vi "Joystick 2 ClimbSystem.vi"(9 "Range of motion":dbl=90.0 format="%#_13g", 10 "Secondary Joystick Buttons":bool[](array[boolean]), 11 "Secondary Joystick Values":dbl[](array[numeric])) -> (2 "Reset Climber Encoder":bool, 3 "Desired Climber Angle":dbl)   [LabVIEW 2018]
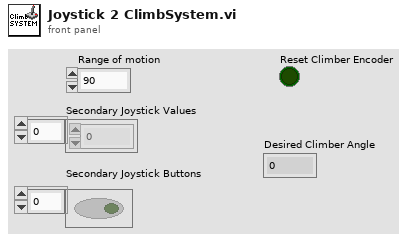
[diagram p1: front panel]
types:
  T1 = typedef "SecondaryJoystickButtons.ctl" = cluster{"Intake":bool, "Outtake":bool, "Arm Up":bool, "Arm Down":bool, "Open Grip":bool, "Close Grip":bool, "Climber Up":bool, "Climber Down":bool, "Reset Climber Encoder":bool}
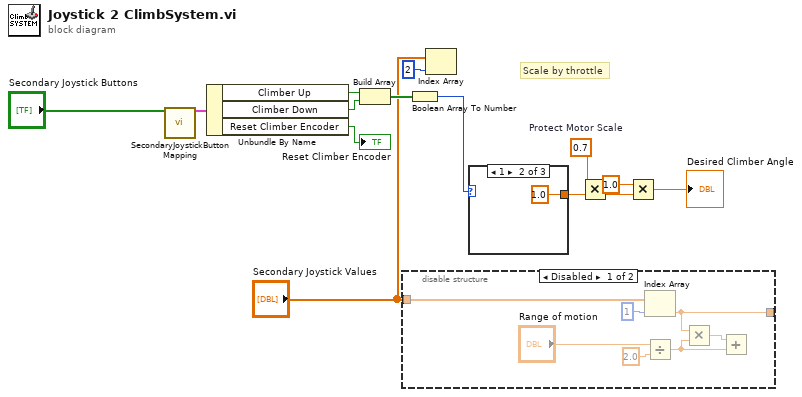
[diagram p0: block diagram]
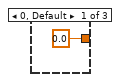
[diagram p2: hidden frame]
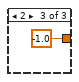
[diagram p3: hidden frame]
diagram:
  w2 = 0.7  # Protect Motor Scale
  # "Scale by throttle"
  n1 = call "SecondaryJoystickButtonMapping.vi"("Secondary joystick buttons"="Secondary Joystick Buttons") -> ("SecondaryJoystickButtons"=w13:T1)  [unwired: 13 in, 1 out]
  n2 = Unbundle By Name(w13) -> ("Climber Up"=w11:bool, "Climber Down"=w10:bool, "Reset Climber Encoder"=→"Reset Climber Encoder":bool)
  n3 = Build Array(w11, w10) -> (w9:bool[])
  n4 = disable-structure shown="Disabled" {
    disable-tunnel: [w16 _] -> _
    disable-tunnel: "Secondary Joystick Values" -> [w15 _]
    frame Disabled {
      n5 = Index Array(array=w15, index=1) -> (element=w16:dbl)
      n6 = Divide(x="Range of motion", y=2.0) -> (x/y=w18:dbl)
      n7 = Multiply(x=w16, y=w18) -> (x*y=w20:dbl)
      n8 = Add(x=w20, y=w18) -> ()  [unwired: 1 out]
    }
    frame Enabled {
    }
  }
  n9 = Boolean Array To Number(Boolean array=w9) -> (number=w8:u32)
  n10 = Index Array(array="Secondary Joystick Values", index=2) -> ()  [unwired: 1 out]
  n11 = case shown="1" w8 {
    tunnel: [0.0 1.0 -1.0] -> w7
    frame 0, Default {
    }
    frame 1 {
    }
    frame 2 {
    }
  }
  n12 = Multiply(x=w2, y=w7) -> (x*y=w3:dbl)
  n13 = Multiply(x=1.0, y=w3) -> (x*y=→"Desired Climber Angle":dbl)
